vi "Filter Available Channels.vi"(11 "DAQmx Shortcuts":T1[](array[typedef])) -> (2 "DAQmx DI Shortcuts":T1[](array[typedef]), 3 "DAQmx AI Shortcuts":T1[](array[typedef]))   [LabVIEW 2019, in "LINX.lvlib" / "LINX.lvclass"]
doc: "Filter all possible DAQmx events down to the global channels configured in MAX."
uses:
  LINX.lvclass
  <resource>/objmgr/daqmx.rc
  LINX Shortcut.ctl
  LINX Channel Type.ctl
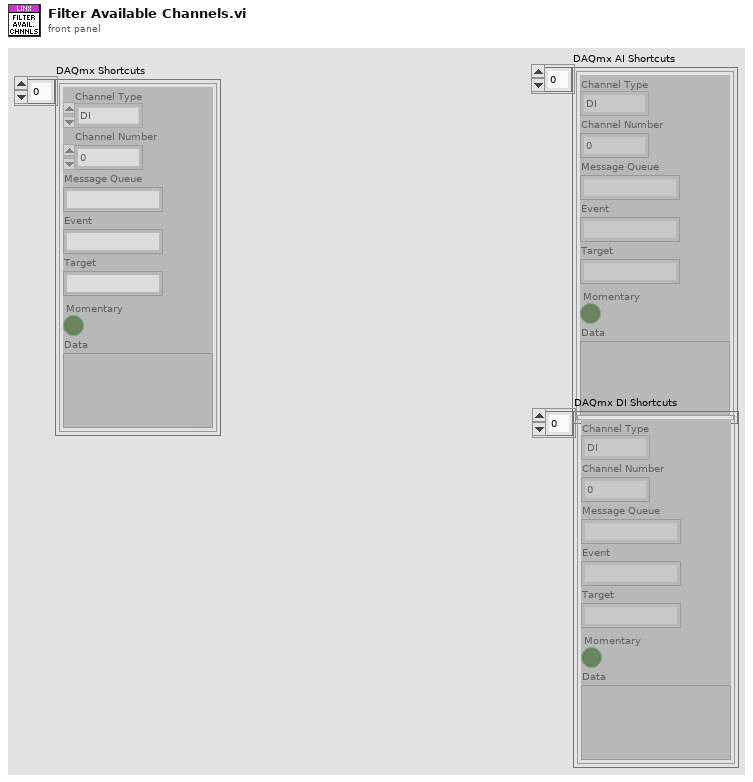
[diagram p1: front panel]
types:
  T1 = typedef "LINX.lvlib/LINX.lvclass/LINX Shortcut.ctl" = cluster{"Channel Type":T2, "Channel Number":u8, "Message Queue":string, "Event":string, "Target":string, "Momentary":bool, "Data":variant}
  T2 = typedef "LINX.lvlib/LINX.lvclass/LINX Channel Type.ctl" = enum16{"DI", "AI"}
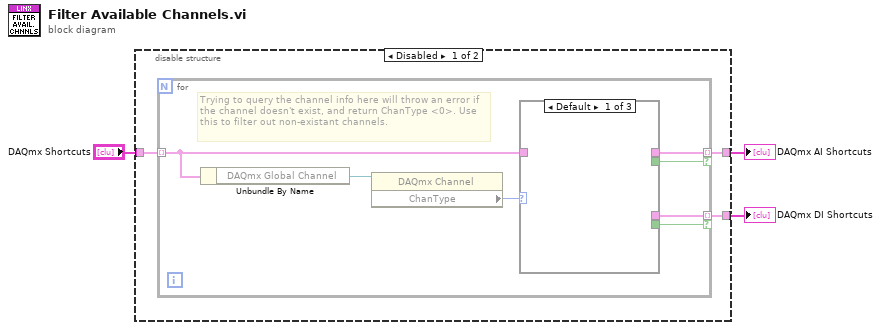
[diagram p0: block diagram]
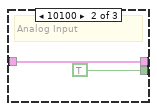
[diagram p2: hidden frame]
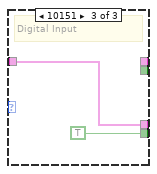
[diagram p3: hidden frame]
diagram:
  n1 = disable-structure shown="Disabled" {
    disable-tunnel: "DAQmx Shortcuts" -> [w6 _]
    disable-tunnel: [w5 _] -> w2
    disable-tunnel: [w4 _] -> w1
    frame Disabled {
      n2 = for {
        tunnel: w6 -> [w11] mode=indexing
        tunnel: [w10] -> w5 mode=indexing if=w8
        tunnel: [w9] -> w4 mode=indexing if=w7
        # "Trying to query the channel info here will throw an error if the channel doesn't exist, and return ChanType <0>. Use this to filter out non-existant channels."
        n3 = Unbundle By Name(w11) -> ("DAQmx Global Channel"=w13:refnum<k21>)
        n4 = property class="DAQmx Channel"(reference=w13) -> ("ChanType"=w12:i32)  [unwired: 1 in, 2 out]
        n5 = case shown="Default" w12 {
          tunnel: w11 -> [_ w15 w17]
          tunnel: [_ w15 _] -> w10
          tunnel: [_ TRUE _] -> w8
          tunnel: [_ _ w17] -> w9
          tunnel: [_ _ TRUE] -> w7
          frame Default {
          }
          frame 10100 {
            # "Analog Input"
          }
          frame 10151 {
            # "Digital Input"
          }
        }
      }
    }
    frame Enabled {
    }
  }
  "DAQmx AI Shortcuts" <- w2
  "DAQmx DI Shortcuts" <- w1
